vi "图像变换.vi"() -> (3 "簇":T1)   [LabVIEW 2018]
panel:
  in  "是否镜像":bool
  in  "镜像方式":u32(ring) items=["Horizontal", "Vertical", "Central", "1st Diagonal", "2nd Diagonal"]
  in  "确认":bool
  in  "旋转角度":dbl
  in  "移动y":dbl
  in  "移动x":dbl
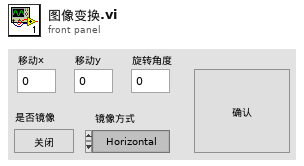
[diagram p1: front panel]
types:
  T1 = cluster{"移动x":dbl, "移动y":dbl, "旋转角度":dbl, "是否镜像":bool, "镜像方法":u32}
  T2 = cluster{"移动x":dbl, "移动y":dbl, "旋转角度":dbl, "是否镜像":bool, "镜像方式":u32}
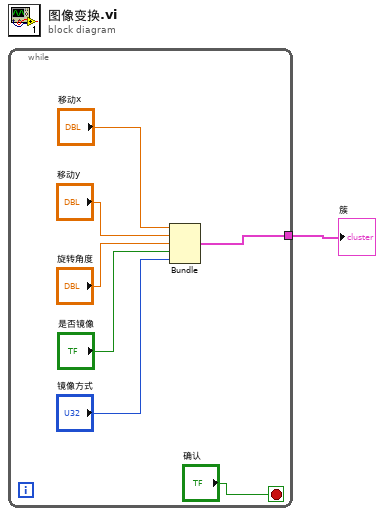
[diagram p0: block diagram]
diagram:
  n1 = while {
    tunnel: [w4] -> w1
    stop <- "确认" stop-if-true
    n2 = Bundle("移动x"="移动x", "移动y"="移动y", "旋转角度"="旋转角度", "是否镜像"="是否镜像", "镜像方式"="镜像方式") -> (w4:T2)  [unwired: 1 in]
  }
  "簇" <- w1
